vi "GetImageTitle.vi"() -> (1 "Error":bool, 2 "Value":string)   [LabVIEW 2014]
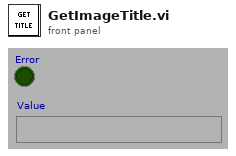
[diagram p1: front panel]
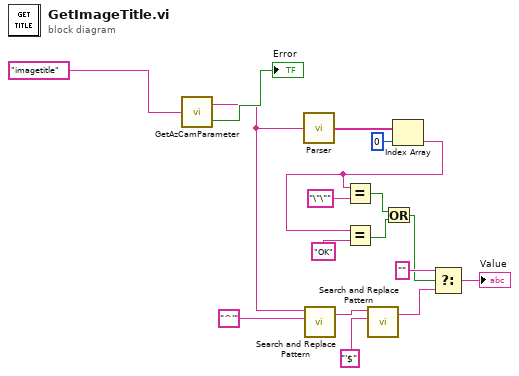
[diagram p0: block diagram]
diagram:
  n1 = call "GetAzCamParameter.vi"("Parameter"="imagetitle" ("Attribute")) -> ("Error"=→"Error":bool, "Value"=w1:string)
  n2 = call "Parser.vi"("string"=w1) -> ("Out Strings"=w16:string[])
  n3 = call <vilib>:"Search and Replace Pattern.vi"("string"=w1, "regular expression (\"\")"="^'" ("regular expression (\"\")")) -> ("result string"=w6:string)  [unwired: 3 in, 1 out]
  n4 = call <vilib>:"Search and Replace Pattern.vi"("string"=w6, "regular expression (\"\")"="'$" ("regular expression (\"\")")) -> ("result string"=w4:string)  [unwired: 3 in, 1 out]
  n5 = Index Array(array=w16, index=0) -> (element=w12:string)
  n6 = Equal?(x=w12, y="\"\"") -> (x = y?=w10:bool)
  n7 = Equal?(x=w12, y="OK") -> (x = y?=w9:bool)
  n8 = Or(x=w10, y=w9) -> (x .or. y?=w8:bool)
  n9 = Select(t="", s=w8, f=w4) -> (s? t:f=→"Value":string)
